vi "Write Timing.vi"(10 "Timing":string="C:\\Sandbox\\Supporting Materials\\Digital\\Timing\\timesets.digitiming", 11 "niDigital in":refnum<class "niDigital.lvclass">) -> (3 "niDigital out":refnum<class "niDigital.lvclass">)   [LabVIEW 2020, in "niDigital.lvclass"]
uses:
  niDigital.lvclass
  niDigital.lvclass/niDigital.ctl
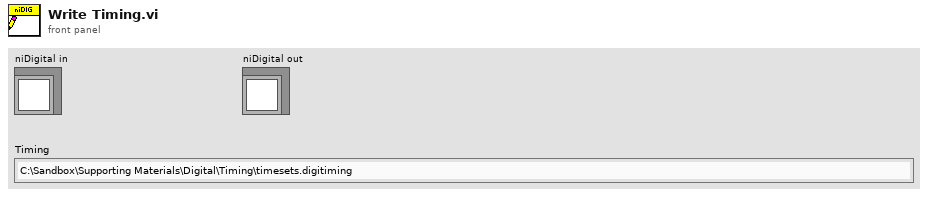
[diagram p1: front panel]
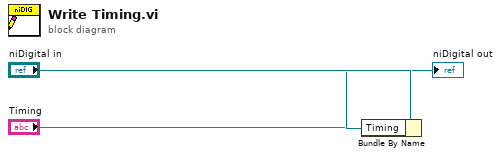
[diagram p0: block diagram]
diagram:
  n1 = Bundle By Name(cluster="niDigital in", "Timing"="Timing") -> (→"niDigital out":refnum<class "niDigital.lvclass">)
